vi "DebugModeSingleton.vi"(7 "Write?":bool, 11 "Debug?":bool) -> (3 "Debug Mode?":bool)   [LabVIEW 2020]
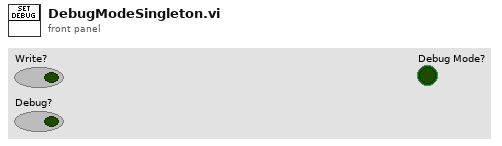
[diagram p1: front panel]
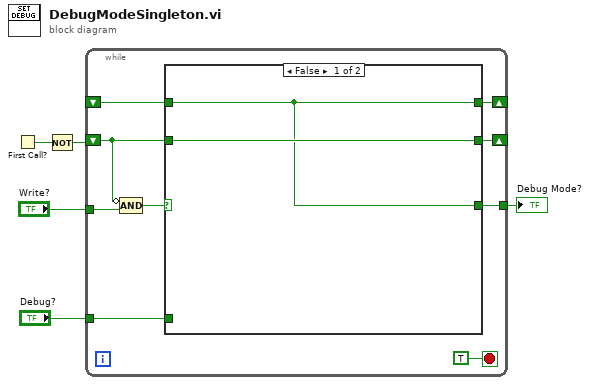
[diagram p0: block diagram]
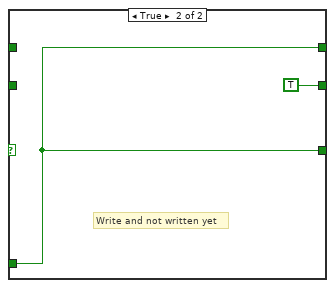
[diagram p2: hidden frame]
diagram:
  n1 = First Call?() -> (First Call?: T/F=w2:bool)
  n2 = Not(x=w2) -> (.not. x?=w1:bool)
  n3 = while {
    tunnel: "Write?" -> [w12]
    shift-right: [w14] -> _
    shift-left: w1 -> [w13]
    tunnel: "Debug?" -> [w9]
    shift-right: [w8] -> _
    shift-left: _ -> [w7]
    tunnel: [w6] -> w3
    stop <- TRUE stop-if-true
    n4 = Compound Arithmetic op=AND(invert w13, w12) -> (w11:bool)
    n5 = case shown="False" w11 {
      tunnel: [w16 TRUE] -> w14
      tunnel: w13 -> [w16 _]
      tunnel: w9 -> [_ w17]
      tunnel: [w15 w17] -> w8
      tunnel: w7 -> [w15 _]
      tunnel: [w15 w17] -> w6
      frame False {
      }
      frame True {
        # "Write and not written yet"
      }
    }
  }
  "Debug Mode?" <- w3
